vi "Init.vi"(11 "Message":T1 {"MessageMetadata"."AbsoluteTime" format="%<%x %.3X>T"}) -> (5 "{{Name}}Message":refnum<class "{{Name}}Message.lvclass">)   [LabVIEW 2020, in "_Template.lvlib" / "Templates.lvlib" / "{{Name}}Message.lvlib" / "{{Name}}Message.lvclass"]
uses:
  {{Name}}Message.lvclass
  {{Name}}Message.lvclass/{{Name}}Message.ctl
  jettl/jettl/ActorRelation.ctl
  jettl/jettl/jettl.lvlib
  jettl/jettl/ActorLifetime.ctl
  jettl/jettl/MessageMetadata.ctl
  Message.ctl
  {{Name}}Message.lvlib
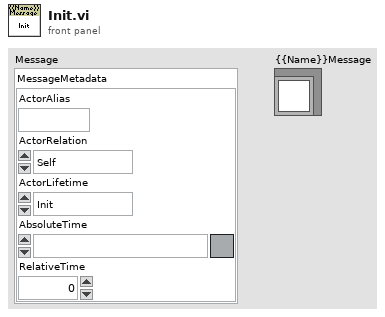
[diagram p1: front panel]
types:
  T1 = typedef "_Template.lvlib/Templates.lvlib/{{Name}}Message.lvlib/Message.ctl" = cluster{"MessageMetadata":T2}
  T2 = typedef "jettl.lvlib/MessageMetadata.ctl" = cluster{"ActorAlias":string, "ActorRelation":T3, "ActorLifetime":T4, "AbsoluteTime":timestamp, "RelativeTime":dbl}
  T3 = typedef "jettl.lvlib/ActorRelation.ctl" = enum16{"Self", "Actor"}
  T4 = typedef "jettl.lvlib/ActorLifetime.ctl" = enum16{"Init", "Spawn", "Setup", "Teardown Before Running", "Running", "Stop Called", "Stopping With Children", "Stopping Without Children", "Teardown After Running", "Stopped"}
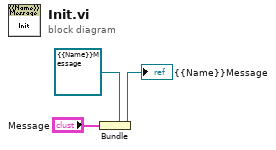
[diagram p0: block diagram]
diagram:
  n1 = Bundle(cluster=refnum<class "{{Name}}Message.lvclass"> refnum ("_Template.lvlib:Templates.lvlib:{{Name}}Message.lvlib:{{Name}}Message.lvclass"), "Message") -> (→"{{Name}}Message":refnum<class "{{Name}}Message.lvclass">)
